vi "Read External Shunt Resistor Value.vi"(8 "error in (no error)":errorcluster, 11 "BNT_DAQmx-MCSV-I in":refnum<class "BNT_DAQmx-MCSV-I.lvclass">) -> (0 "error out":errorcluster, 2 "External Shunt Resistor Value":dbl[unit]=249.0 format="%0.2f", 3 "BNT_DAQmx-MCSV-I out":refnum<class "BNT_DAQmx-MCSV-I.lvclass">)   [LabVIEW 2020, in "BNT_DAQmx.lvlib" / "BNT_DAQmx-MCSV-I.lvclass"]
doc: "Read external shunt resistor value."
uses:
  BNT_DAQmx-MCSV-I.lvclass
  BNT_DAQmx-MCSV-I.lvclass/BNT_DAQmx-MCSV-I.ctl
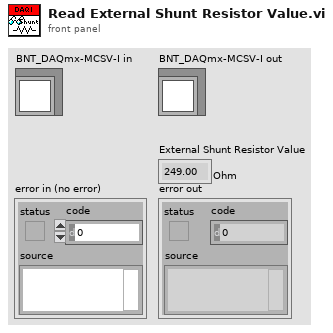
[diagram p1: front panel]
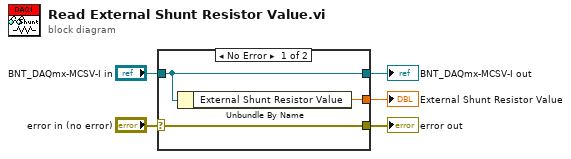
[diagram p0: block diagram]
diagram:
  n1 = case shown="No Error" "error in (no error)" {
    selector: "error in (no error)" -> [w8 w9]
    tunnel: [w8 w9] -> w4
    tunnel: [w7 w10] -> w2
    tunnel: "BNT_DAQmx-MCSV-I in" -> [w7 w10]
    tunnel: [w6 _] -> w1
    frame No Error {
      n2 = Unbundle By Name(w7) -> ("External Shunt Resistor Value"=w6:dbl[unit])
    }
    frame Error {
    }
  }
  "error out" <- w4
  "BNT_DAQmx-MCSV-I out" <- w2
  "External Shunt Resistor Value" <- w1
